vi "Initialize all mailboxes.vi"(8 "error in (no error)":errorcluster, 11 "MailboxSize(-1)":i32=-1) -> (0 "error out":errorcluster, 3 "Referencies out":T1)   [LabVIEW 2021, in "MessengerLib.lvlib"]
uses:
  MessengerLib.lvlib
  Data types/Messenger referencies.ctl
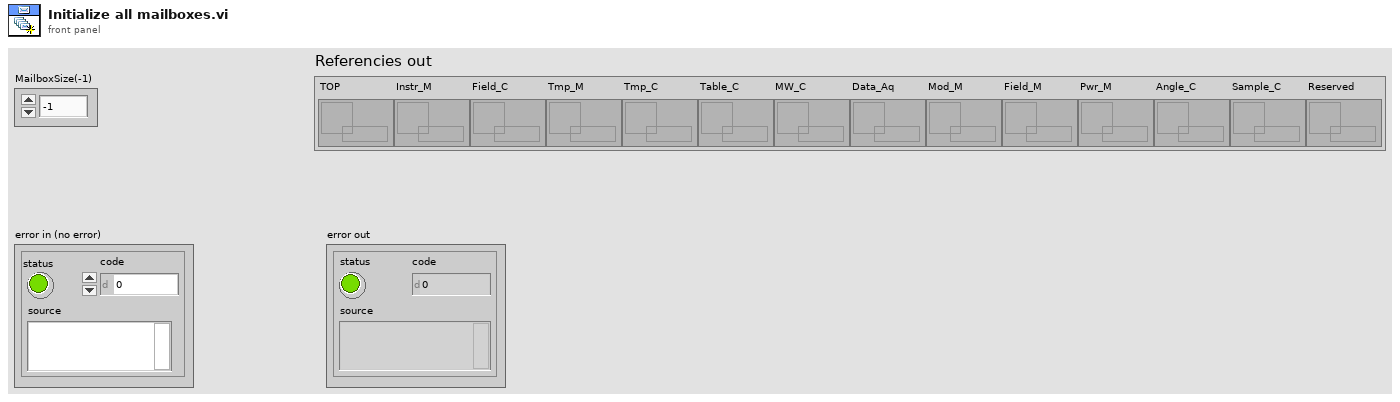
[diagram p1: front panel]
types:
  T1 = typedef "MessengerLib.lvlib/Messenger referencies.ctl" = cluster{"TOP":refnum<queue>, "Instr_M":refnum<queue>, "Field_C":refnum<queue>, "Tmp_M":refnum<queue>, "Tmp_C":refnum<queue>, "Table_C":refnum<queue>, "MW_C":refnum<queue>, "Data_Aq":refnum<queue>, "Mod_M":refnum<queue>, "Field_M":refnum<queue>, "Pwr_M":refnum<queue>, "Angle_C":refnum<queue>, "Sample_C":refnum<queue>, "Reserved":refnum<queue>}
  T2 = cluster{"[0]":refnum<queue>, "[1]":refnum<queue>, "[2]":refnum<queue>, "[3]":refnum<queue>, "[4]":refnum<queue>, "[5]":refnum<queue>, "[6]":refnum<queue>, "[7]":refnum<queue>, "[8]":refnum<queue>, "[9]":refnum<queue>, "[10]":refnum<queue>, "[11]":refnum<queue>, "[12]":refnum<queue>, "[13]":refnum<queue>}
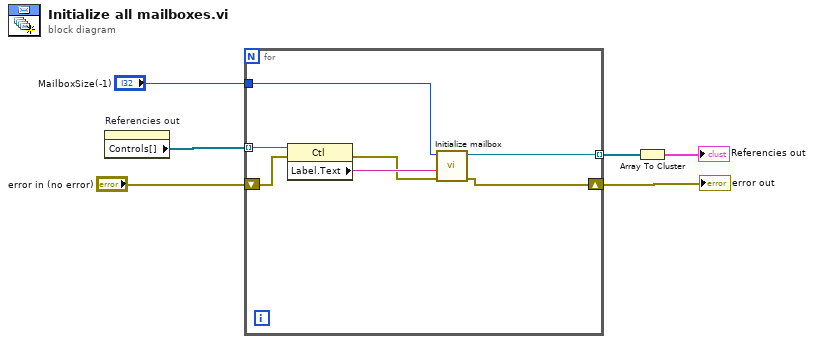
[diagram p0: block diagram]
diagram:
  n1 = property on="Referencies out" class="Clust (strict)"() -> ("Controls[]"=w3:refnum<vi>[])  [unwired: 2 in, 2 out]
  n2 = for {
    tunnel: w3 -> [w13] mode=indexing
    tunnel: [w10] -> w4 mode=indexing
    shift-right: [w9] -> w6
    shift-left: "error in (no error)" -> [w8]
    tunnel: "MailboxSize(-1)" -> [w7]
    n3 = property class="Ctl"(reference=w13, error in=w8) -> (error out=w11:errorcluster, "Label.Text"=w12:string)  [unwired: 1 out]
    n4 = call "Initialize mailbox.vi"("error in"=w11, "name (unnamed)"=w12, "MailboxSize(-1)"=w7) -> ("error out"=w9:errorcluster, "Queue out"=w10:refnum<queue>)  [unwired: 7 in]
  }
  "error out" <- w6
  n5 = Array To Cluster(array=w4) -> (cluster=→"Referencies out":T2)
